vi "DB and RH to WB.vi"(1 "Relative Humidity [%]":dbl, 2 "Dry Bulb Temp [DegF]":dbl) -> (0 "Wet Bulb Temp [DegF]":dbl)   [LabVIEW 2020]
panel:
  # "https://www.omnicalculator.com/physics/wet-bulb"
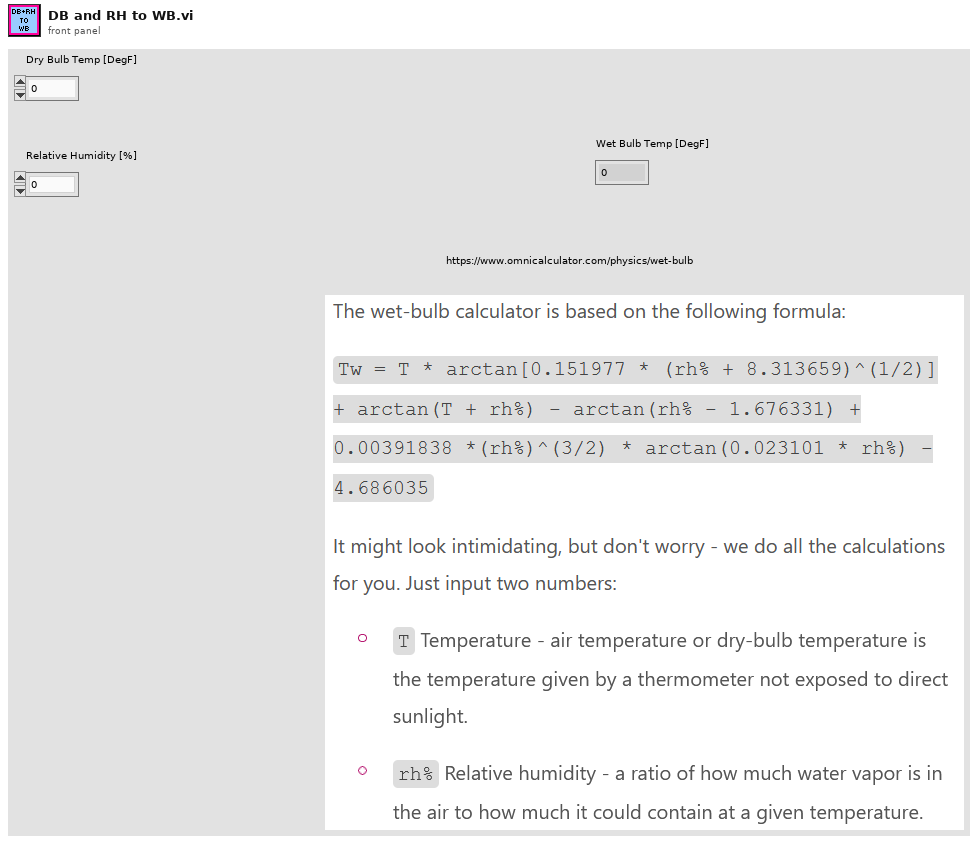
[diagram p1: front panel]
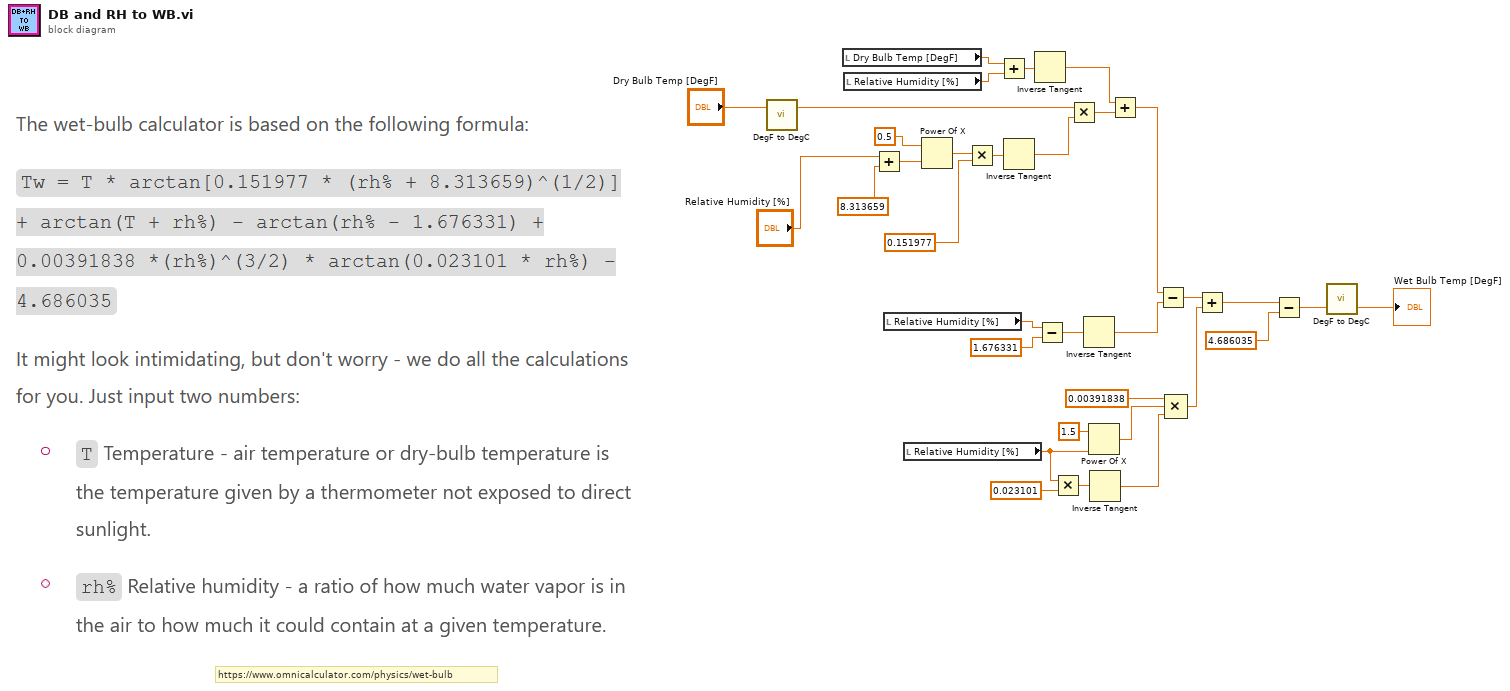
[diagram p0: block diagram]
diagram:
  # "https://www.omnicalculator.com/physics/wet-bulb"
  n1 = call "DegF to DegC.vi"("Input Temperature in Fahrenheit"="Dry Bulb Temp [DegF]") -> ("Output Temperature in Celcius"=w3:dbl)  [unwired: 1 in, 1 out]
  n2 = local read "Dry Bulb Temp [DegF]"() -> (w24:dbl)
  n3 = local read "Relative Humidity [%]"() -> (w23:dbl)
  n4 = Add(x="Relative Humidity [%]", y=8.313659) -> (x+y=w26:dbl)
  n5 = local read "Relative Humidity [%]"() -> (w20:dbl)
  n6 = local read "Relative Humidity [%]"() -> (w10:dbl)
  n7 = Power Of X(1:w26, 2:0.5 ("x")) -> (0:w31:dbl)
  n8 = Multiply(x=w31, y=0.151977) -> (x*y=w29:dbl)
  n9 = Add(x=w24, y=w23) -> (x+y=w22:dbl)
  n10 = Inverse Tangent(1:w29) -> (0:w28:dbl)
  n11 = Inverse Tangent(1:w22) -> (0:w21:dbl)
  n12 = Subtract(x=w20, y=1.676331) -> (x-y=w18:dbl)
  n13 = Multiply(x=w10, y=0.023101) -> (x*y=w11:dbl)
  n14 = Multiply(x=w3, y=w28) -> (x*y=w25:dbl)
  n15 = Inverse Tangent(1:w18) -> (0:w6:dbl)
  n16 = Power Of X(1:w10, 2:1.5 ("y")) -> (0:w13:dbl)
  n17 = Inverse Tangent(1:w11) -> (0:w12:dbl)
  n18 = Add(x=w21, y=w25) -> (x+y=w5:dbl)
  n19 = Subtract(x=w5, y=w6) -> (x-y=w17:dbl)
  n20 = Compound Arithmetic op=MULTIPLY(0.00391838 ("value"), w13, w12) -> (w16:dbl)
  n21 = Add(x=w17, y=w16) -> (x+y=w8:dbl)
  n22 = Subtract(x=w8, y=4.686035) -> (x-y=w2:dbl)
  n23 = call "DegF to DegC.vi"("Input Temperature in Celcius"=w2) -> ("Output Temperature in Fahrenheit"=→"Wet Bulb Temp [DegF]":dbl)  [unwired: 1 in, 1 out]
